vi "ConvertToU8.vi"(1 "struct":string="\"<BBI\", __USBDBG_CMD, __USBDBG_SCRIPT_EXEC, 27") -> (0 "Binary":string)   [LabVIEW 2022 SP3]
uses:
  <vilib>/Utility/error.llb/Trim Whitespace One-Sided.vi
panel:
  out "Array":u8[](array[numeric])=[48, 5, 27, 0, 0, 0] format="%.0x"
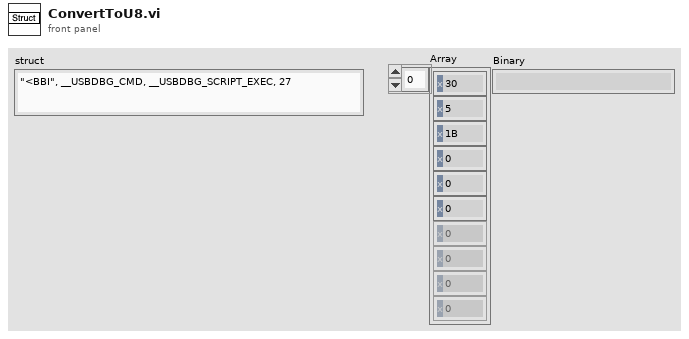
[diagram p1: front panel]
types:
  T1 = enum16{"big-endian, network order", "native, host order", "little-endian"}
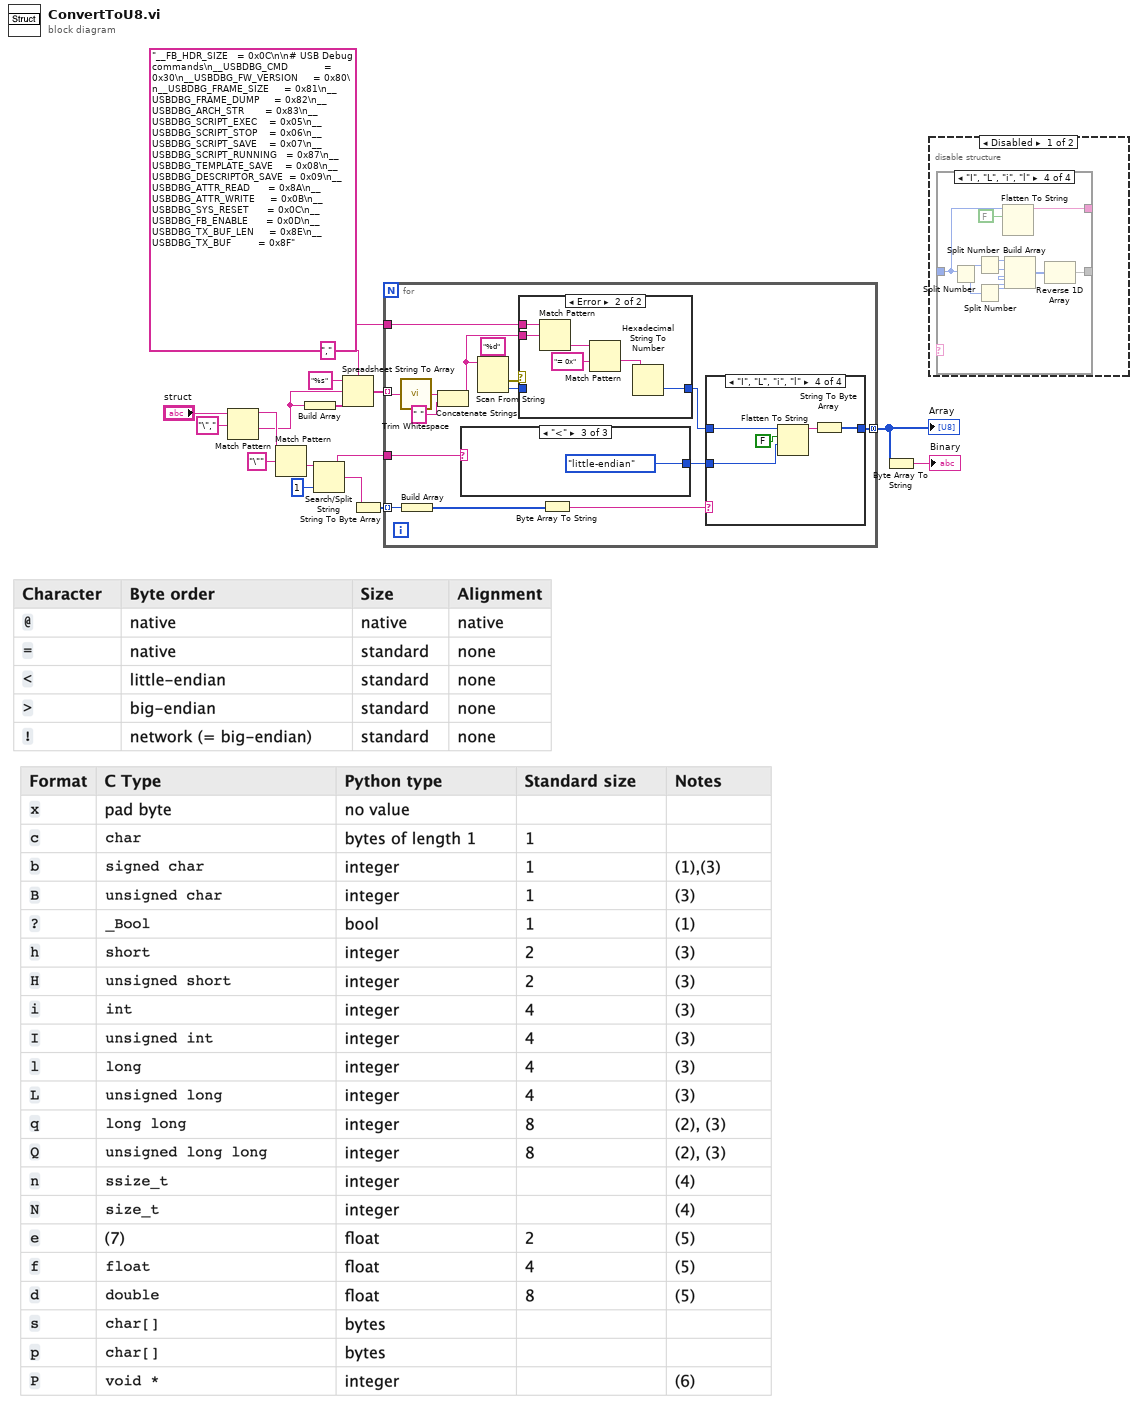
[diagram p0: block diagram]
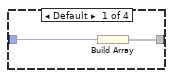
[diagram p2: hidden frame]
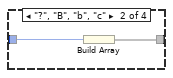
[diagram p3: hidden frame]
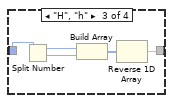
[diagram p4: hidden frame]
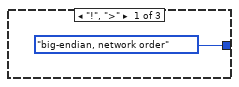
[diagram p6: hidden frame]
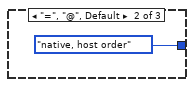
[diagram p7: hidden frame]
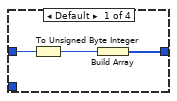
[diagram p9: hidden frame]
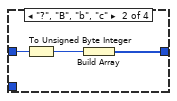
[diagram p10: hidden frame]
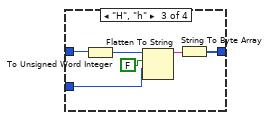
[diagram p11: hidden frame]
diagram:
  n1 = Match Pattern(string="struct", regular expression="\",") -> (before substring=w16:string, after substring=w7:string)  [unwired: 1 in, 2 out]
  n2 = Match Pattern(string=w16, regular expression="\"") -> (after substring=w4:string)  [unwired: 1 in, 3 out]
  n3 = Build Array(w7) -> (w13:string[])
  n4 = Search/Split String(string=w4, offset (0)=1) -> (substring before match=w1:string, match + rest of string=w3:string)  [unwired: 1 in, 1 out]
  n5 = Spreadsheet String To Array(delimiter (Tab)=",", format string="%s", spreadsheet string=w7, array type (2D Dbl)=w13) -> (array=w10:string[])
  n6 = String To Byte Array(string=w3) -> (unsigned byte array=w14:u8[])
  n7 = for {
    tunnel: w14 -> [w32] mode=indexing
    tunnel: w10 -> [w26] mode=indexing
    tunnel: "__FB_HDR_SIZE   = 0x0C\n\n# USB Debug commands\n__USBDBG_CMD            = 0x30\n__USBDBG_FW_VERSION     = 0x80\n__USBDBG_FRAME_SIZE     = 0x81\n__USBDBG_FRAME_DUMP     = 0x82\n__USBDBG_ARCH_STR       = 0x83\n__USBDBG_SCRIPT_EXEC    = 0x05\n__USBDBG_SCRIPT_STOP    = 0x06\n__USBDBG_SCRIPT_SAVE    = 0x07\n__USBDBG_SCRIPT_RUNNING   = 0x87\n__USBDBG_TEMPLATE_SAVE    = 0x08\n__USBDBG_DESCRIPTOR_SAVE  = 0x09\n__USBDBG_ATTR_READ      = 0x8A\n__USBDBG_ATTR_WRITE     = 0x0B\n__USBDBG_SYS_RESET      = 0x0C\n__USBDBG_FB_ENABLE      = 0x0D\n__USBDBG_TX_BUF_LEN     = 0x8E\n__USBDBG_TX_BUF         = 0x8F" ("Constants") -> [w29]
    tunnel: [w27] -> w6 mode=concatenating
    tunnel: w1 -> [w22]
    n8 = call <vilib>:"Trim Whitespace.vi"("string"=w26) -> ("trimmed string"=w20:string)  [unwired: 1 in]
    n9 = Build Array(w32) -> (w31:u8[])
    n10 = Concatenate Strings(w20, " " ("string")) -> (w18:string)
    n11 = case shown="\"<\"" w22 {
      tunnel: [T1."big-endian, network order" ("byte order (0:big-endian, network order)") T1."native, host order" ("byte order (0:big-endian, network order)") T1."little-endian" ("byte order (0:big-endian, network order)")] -> w21
      frame "!", ">" {
      }
      frame "=", "@", Default {
      }
      frame "<" {
      }
    }
    n12 = Scan From String(format string="%d", input string=w18) -> (error out=w25:errorcluster, output 1=w23:i32)  [unwired: 3 in, 2 out]
    n13 = case shown="Error" w25 {
      tunnel: w29 -> [_ w42]
      tunnel: [w36 w39] -> w28
      tunnel: w18 -> [_ w37]
      tunnel: w23 -> [w36 _]
      frame No Error {
      }
      frame Error {
        n14 = Match Pattern(string=w42, regular expression=w37) -> (after substring=w41:string)  [unwired: 1 in, 3 out]
        n15 = Match Pattern(string=w41, regular expression="= 0x") -> (after substring=w38:string)  [unwired: 1 in, 3 out]
        n16 = Hexadecimal String To Number(string=w38) -> (number=w39:u32)  [unwired: 2 in, 1 out]
      }
    }
    n17 = Byte Array To String(unsigned byte array=w31) -> (string=w30:string)
    n18 = case shown="\"I\", \"L\", \"i\", \"l\"" w30 {
      tunnel: w28 -> [w45 w48 w51 w55]
      tunnel: [w44 w47 w50 w57] -> w27
      tunnel: w21 -> [_ _ w49 w56]
      frame Default {
        n19 = To Unsigned Byte Integer(number=w45) -> (unsigned 8bit integer=w43:u8)
        n20 = Build Array(w43) -> (w44:u8[])
      }
      frame "?", "B", "b", "c" {
        n21 = To Unsigned Byte Integer(number=w48) -> (unsigned 8bit integer=w46:u8)
        n22 = Build Array(w46) -> (w47:u8[])
      }
      frame "H", "h" {
        n23 = To Unsigned Word Integer(number=w51) -> (unsigned 16bit integer=w52:u16)
        n24 = Flatten To String(anything=w52, prepend array or string size? (T)=FALSE, byte order (0:big-endian, network order)=w49) -> (data string=w53:string)  [unwired: 1 in, 2 out]
        n25 = String To Byte Array(string=w53) -> (unsigned byte array=w50:u8[])
      }
      frame "I", "L", "i", "l" {
        n26 = Flatten To String(anything=w55, prepend array or string size? (T)=FALSE, byte order (0:big-endian, network order)=w56) -> (data string=w58:string)  [unwired: 1 in, 2 out]
        n27 = String To Byte Array(string=w58) -> (unsigned byte array=w57:u8[])
      }
    }
  }
  "Array" <- w6
  n28 = Byte Array To String(unsigned byte array=w6) -> (string=→"Binary":string)
  n29 = disable-structure shown="Disabled" {
    frame Disabled {
      n30 = case shown="\"I\", \"L\", \"i\", \"l\"" {
        selector: _ -> [_ _ _ _]
        tunnel: _ -> [w61 w63 w68 w71]
        tunnel: [w60 w62 w64 w78] -> _
        tunnel: [_ _ _ w69] -> _
        frame Default {
          n31 = Build Array(w61) -> (w60:void[])
        }
        frame "?", "B", "b", "c" {
          n32 = Build Array(w63) -> (w62:void[])
        }
        frame "H", "h" {
          n33 = Split Number(x=w68) -> (hi(x)=w67:u16, lo(x)=w66:u16)
          n34 = Build Array(w67, w66) -> (w65:u16[])
          n35 = Reverse 1D Array(array=w65) -> (reversed array=w64:u16[])
        }
        frame "I", "L", "i", "l" {
          n36 = Split Number(x=w71) -> (hi(x)=w77:u16, lo(x)=w76:u16)
          n37 = Split Number(x=w77) -> (hi(x)=w74:u8, lo(x)=w75:u8)
          n38 = Split Number(x=w76) -> (hi(x)=w73:u8, lo(x)=w72:u8)
          n39 = Flatten To String(anything=w71, prepend array or string size? (T)=FALSE) -> (data string=w69:string)  [unwired: 2 in, 2 out]
          n40 = Build Array(w74, w75, w73, w72) -> (w79:u8[])
          n41 = Reverse 1D Array(array=w79) -> (reversed array=w78:u8[])
        }
      }
    }
    frame Enabled {
    }
  }
